vi "Define.vi"() -> (3 "ID out":refnum<class "ID.lvclass">)   [LabVIEW 2020, in "Conditu2.lvlib" / "Columns.lvlib" / "ID.lvclass"]
uses:
  ID.lvclass
  C:/dev/lv20CE/lv-conditum-tools/Conditum-Clone/Columns/Type/Type.lvclass
  Type/Definition.ctl
  Attributes.ctl
  Field Type.ctl
  Type/Type.lvclass/Type.ctl
  Type/Type.lvclass
  Conditu2.lvlib
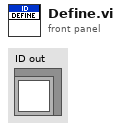
[diagram p1: front panel]
types:
  T1 = typedef "Conditu2.lvlib/Field Type.ctl" = enum16{"None", "ID", "Boolean", "Integer", "Double", "Timestamp", "String", "Text", "Entity"}
  T2 = typedef "Conditu2.lvlib/Attributes.ctl" = cluster{"Primary Key":bool, "Unique":bool, "Foreign Key":bool, "Auto Increment":bool}
  T3 = typedef "Conditu2.lvlib/Columns.lvlib/Type.lvclass/Definition.ctl" = cluster{"Name":string, "Nullable":bool, "Default NULL":bool}
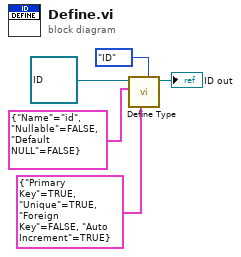
[diagram p0: block diagram]
diagram:
  n1 = call "Define Type.vi"("Type"=Field_Type."ID", "Attributes"=T2 {"Primary Key"=TRUE, "Unique"=TRUE, "Foreign Key"=FALSE, "Auto Increment"=TRUE}, "Definition"=T3 {"Name"="id", "Nullable"=FALSE, "Default NULL"=FALSE}, "Type in"=refnum<class "ID.lvclass"> refnum ("ID out")) -> ("Type out"=→"ID out":refnum<class "ID.lvclass">)  [unwired: 7 in]
